vi "Simple - File Input.vi"() -> ()   [LabVIEW 2018]
doc: "Demonstrates compiling a logic-free mustache template stored in a file. Only variable tags are used in this example."
uses:
  Toolkit/Support/Compile with String Array.vi
  Toolkit/Toolkit.lvlib
panel:
  in  "Input":path
  in  "Data":cluster{"Key":string, "Value":string}[](array[cluster])=[{"Key"="greeting", "Value"="Hello"}, {"Key"="name", "Value"="World"}]
  out "Output":string
  # "Overview: Demonstrates compiling a mustache template string with only variable tags\nInstructions:\n1. Select a Mustache template file (*.mustache) that only has variable tags, or leave the Input control blank to use the default Mustache template file provided with this example.\n2. Enter the key-value pair data for each of the variable tags\n3. Run the VI"
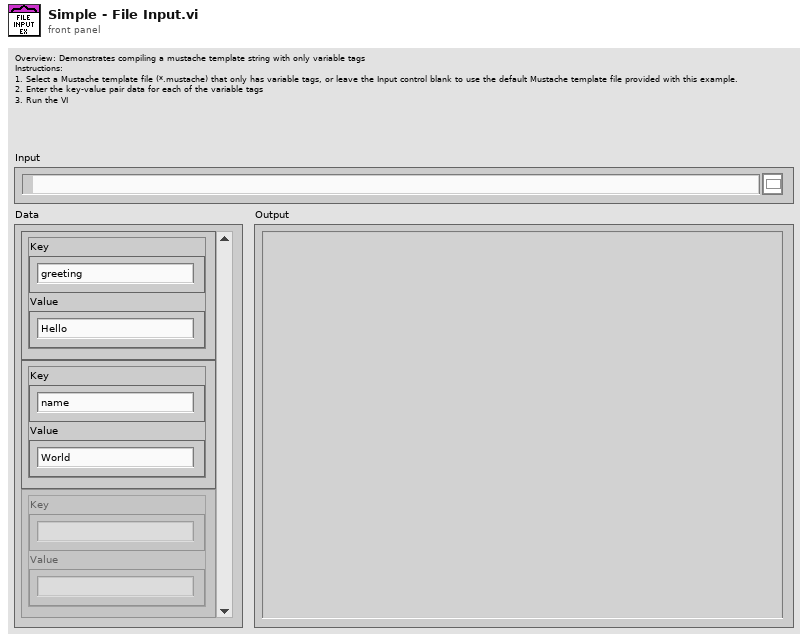
[diagram p1: front panel]
types:
  T1 = enum16{"open", "replace", "create", "open or create", "replace or create", "replace or create with confirmation"}
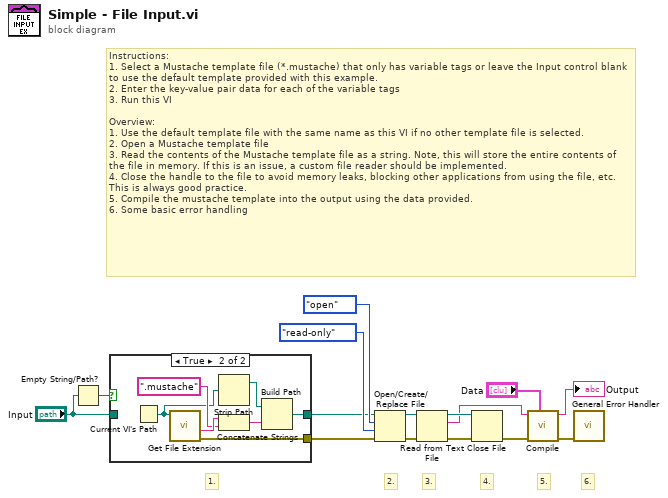
[diagram p0: block diagram]
diagram:
  # "6."
  # "5."
  # "4."
  # "3."
  # "2."
  # "1."
  # "Instructions:\n1. Select a Mustache template file (*.mustache) that only has variable tags or leave the Input control blank to use the default template provided with this example.\n2. Enter the key-value pair data for each of the variable tags\n3. Run this VI \n\nOverview:\n1. Use the default template file with the same name as this VI if no other template file is selected.\n2. Open a Mustache template file\n3. Read the contents of the Mustache template file as a string. Note, this will store the entire contents of the file in memory. If this is an issue, a custom file reader should be implemented.\n4. Close the handle to the file to avoid memory leaks, blocking other applications from using the file, etc. This is always good practice.\n5. Compile the mustache template into the output using the data provided.\n6. Some basic error handling"
  n1 = Empty String/Path?(string/path="Input") -> (empty?=w9:bool)
  n2 = case shown="True" w9 {
    tunnel: [w16 w18] -> w8
    tunnel: "Input" -> [w16 _]
    tunnel: [_ w17] -> w6
    frame False {
    }
    frame True {
      n3 = Current VI's Path() -> (path=w21:path)
      n4 = call <vilib>:"Get File Extension.vi"("file"=w21) -> ("error out"=w17:errorcluster, "filename without extension"=w23:string)  [unwired: 6 in, 3 out]
      n5 = Strip Path(path=w21) -> (stripped path=w20:path)  [unwired: 1 out]
      n6 = Concatenate Strings(w23, ".mustache" ("string")) -> (w19:string)
      n7 = Build Path(base path=w20, name or relative path=w19) -> (appended path=w18:path)
    }
  }
  n8 = Open/Create/Replace File(file path (use dialog)=w8, error in=w6, operation (0:open)=T1."open", access (0:read/write)=enum16{"read/write", "read-only", "write-only"}."read-only") -> (refnum out=w15:refnum<file>, error out=w14:errorcluster)  [unwired: 2 in, 1 out]
  n9 = Read from Text File(file (use dialog)=w15, error in=w14) -> (refnum out=w13:refnum<file>, text=w1:string, error out=w12:errorcluster)  [unwired: 2 in, 1 out]
  n10 = Close File(refnum=w13, error in=w12) -> (error out=w2:errorcluster)  [unwired: 1 out]
  n11 = call-poly "Compile.vi"("Data"="Data", "Error In"=w2, "Input"=w1) -> ("Error Out"=w3:errorcluster, "Output"=→"Output":string)  [unwired: 7 in]
  n12 = call <vilib>:"General Error Handler.vi"("error in (no error)"=w3) -> ()  [unwired: 10 in, 5 out]
